vi "test_read-nmea-data2.vi"() -> ()   [LabVIEW 2019] (continued)
,E,2.703,238.94,250720,,,A,V*0C\n\t\n15:14:55.25\tF9P\t$GNVTG,238.94,T,,M,2.703,N,5.005,K,A*21\n\t\n15:14:55.27\tF9P\t$GNGGA,061457.00,3723.60262,N,12656.95923,E,1,12,0.72,45.1,M,18.5,M,,*7E\n\t\n15:14:55.29\tF9P\t$GNGSA,A,3,12,06,19,05,17,09,04,02,,,,,1.24,0.72,1.01,1*02\n\t\n15:14:55.31\tF9P\t$GNGSA,A,3,85,70,71,84,,,,,,,,,1.24,0.72,1.01,2*00\n\t\n15:14:55.33\tF9P\t$GNGSA,A,3,36,19,11,04,09,12,,,,,,,1.24,0.72,1.01,3*02\n\t\n15:14:55.35\tF9P\t$GNGSA,A,3,14,11,33,,,,,,,,,,1.24,0.72,1.01,4*03\n\t\n15:14:55.37\tF9P\t$GPGSV,3,1,09,02,56,320,27,04,17,043,29,05,38,248,35,06,64,051,32,1*63\n\t\n15:14:55.39\tF9P\t$GPGSV,3,2,09,09,44,072,37,12,23,275,25,17,32,154,28,19,51,157,26,1*67\n\t\n15:14:55.41\tF9P\t$GPGSV,3,3,09,25,12,306,15,1*58\n\t\n15:14:55.43\tF9P\t$GPGSV,3,1,09,02,56,320,,04,17,043,19,05,38,248,28,06,64,051,28,6*65\n\t\n15:14:55.45\tF9P\t$GPGSV,3,2,09,09,44,072,29,12,23,275,18,17,32,154,17,19,51,157,,6*69\n\t\n15:14:55.47\tF9P\t$GPGSV,3,3,09,25,12,306,,6*5B\n\t\n15:14:55.49\tF9P\t$GLGSV,2,1,08,69,10,031,30,70,70,037,33,71,54,207,34,72,05,210,,1*7E\n\t\n15:14:55.51\tF9P\t$GLGSV,2,2,08,77,01,324,,84,19,123,18,85,69,072,42,86,38,331,,1*7C\n\t\n15:14:55.53\tF9P\t$GLGSV,2,1,08,69,10,031,19,70,70,037,,71,54,207,30,72,05,210,,3*73\n\t\n15:14:55.55\tF9P\t$GLGSV,2,2,08,77,01,324,,84,19,123,21,85,69,072,24,86,38,331,,3*74\n\t\n15:14:55.57\tF9P\t$GAGSV,2,1,08,02,08,296,09,04,67,115,32,09,33,193,26,11,72,001,25,7*72\n\t\n15:14:55.59\tF9P\t$GAGSV,2,2,08,12,39,103,32,19,25,045,34,25,08,248,14,36,27,309,19,7*7E\n\t\n15:14:55.61\tF9P\t$GAGSV,2,1,08,02,08,296,,04,67,115,,09,33,193,,11,72,001,,2*7C\n\t\n15:14:55.63\tF9P\t$GAGSV,2,2,08,12,39,103,,19,25,045,,25,08,248,,36,27,309,,2*70\n\t\n15:14:55.65\tF9P\t$GBGSV,2,1,06,07,,,26,11,48,133,26,14,87,101,30,28,,,23,1*7B\n\t\n15:14:55.67\tF9P\t$GBGSV,2,2,06,33,62,220,33,34,,,25,1*44\n\t\n15:14:55.69\tF9P\t$GBGSV,1,1,03,11,48,133,,14,87,101,30,33,62,220,,3*47\n\t\n15:14:55.71\tF9P\t$GNGLL,3723.60262,N,12656.95923,E,061457.00,A,A*71\n\t\n15:14:55.73\tF9P\t\t\n15:14:55.75\tF9P\t\t\n15:14:55.77\tF9P\t\t\n15:14:55.79\tF9P\t\t\n15:14:55.81\tF9P\t\t\n15:14:55.83\tF9P\t\t\n15:14:55.85\tF9P\t\t\n15:14:55.87\tF9P\t\t\n15:14:55.89\tF9P\t\t\n15:14:55.91\tF9P\t\t\n15:14:55.93\tF9P\t\t\n15:14:55.95\tF9P\t\t\n15:14:55.97\tF9P\t\t\n15:14:55.99\tF9P\t\t\n15:14:56.01\tF9P\t\t\n15:14:56.03\tF9P\t\t\n15:14:56.05\tF9P\t\t\n15:14:56.07\tF9P\t\t\n15:14:56.09\tF9P\t\t\n15:14:56.11\tF9P\t\t\n15:14:56.13\tF9P\t\t\n15:14:56.15\tF9P\t\t\n15:14:56.17\tF9P\t\t\n15:14:56.19\tF9P\t\t\n15:14:56.21\tF9P\t\t\n15:14:56.23\tF9P\t$GNRMC,061458.00,A,3723.60230,N,12656.95830,E,2.766,236.10,250720,,,A,V*06\n\t\n15:14:56.25\tF9P\t$GNVTG,236.10,T,,M,2.766,N,5.123,K,A*25\n\t\n15:14:56.27\tF9P\t$GNGGA,061458.00,3723.60230,N,12656.95830,E,1,12,0.72,45.0,M,18.5,M,,*74\n\t\n15:14:56.29\tF9P\t$GNGSA,A,3,12,06,19,05,17,09,04,02,,,,,1.24,0.72,1.01,1*02\n\t\n15:14:56.31\tF9P\t$GNGSA,A,3,85,70,71,84,,,,,,,,,1.24,0.72,1.01,2*00\n\t\n15:14:56.33\tF9P\t$GNGSA,A,3,36,19,11,04,09,12,,,,,,,1.24,0.72,1.01,3*02\n\t\n15:14:56.35\tF9P\t$GNGSA,A,3,14,11,33,,,,,,,,,,1.24,0.72,1.01,4*03\n\t\n15:14:56.37\tF9P\t$GPGSV,3,1,09,02,56,320,25,04,17,043,28,05,38,248,36,06,64,051,28,1*68\n\t\n15:14:56.39\tF9P\t$GPGSV,3,2,09,09,44,072,38,12,23,275,24,17,32,154,27,19,51,157,26,1*66\n\t\n15:14:56.41\tF9P\t$GPGSV,3,3,09,25,12,306,14,1*59\n\t\n15:14:56.43\tF9P\t$GPGSV,3,1,09,02,56,320,,04,17,043,19,05,38,248,32,06,64,051,33,6*64\n\t\n15:14:56.45\tF9P\t$GPGSV,3,2,09,09,44,072,29,12,23,275,17,17,32,154,16,19,51,157,,6*67\n\t\n15:14:56.47\tF9P\t$GPGSV,3,3,09,25,12,306,,6*5B\n\t\n15:14:56.49\tF9P\t$GLGSV,2,1,08,69,10,031,23,70,70,037,31,71,54,207,32,72,05,210,,1*78\n\t\n15:14:56.51\tF9P\t$GLGSV,2,2,08,77,01,324,,84,19,123,16,85,69,072,43,86,38,331,,1*73\n\t\n15:14:56.53\tF9P\t$GLGSV,2,1,08,69,10,031,18,70,70,037,,71,54,207,28,72,05,210,,3*7B\n\t\n15:14:56.55\tF9P\t$GLGSV,2,2,08,77,01,324,,84,19,123,19,85,69,072,24,86,38,331,,3*7F\n\t\n15:14:56.57\tF9P\t$GAGSV,2,1,08,02,08,296,09,04,67,115,34,09,33,193,25,11,72,001,25,7*77\n\t\n15:14:56.59\tF9P\t$GAGSV,2,2,08,12,39,103,33,19,25,045,37,25,08,248,15,36,27,309,21,7*76\n\t\n15:14:56.61\tF9P\t$GAGSV,2,1,08,02,08,296,,04,67,115,,09,33,193,,11,72,001,,2*7C\n\t\n15:14:56.63\tF9P\t$GAGSV,2,2,08,12,39,103,,19,25,045,,25,08,248,,36,27,309,,2*70\n\t\n15:14:56.65\tF9P\t$GBGSV,2,1,06,07,,,25,11,48,133,26,14,87,101,29,28,,,22,1*71\n\t\n15:14:56.67\tF9P\t$GBGSV,2,2,06,33,62,220,30,34,,,24,1*46\n\t\n15:14:56.69\tF9P\t$GBGSV,1,1,03,11,48,133,,14,87,101,31,33,62,220,,3*46\n\t\n15:14:56.71\tF9P\t$GNGLL,3723.60230,N,12656.95830,E,061458.00,A,A*7A\n\t\n15:14:56.73\tF9P\t\t\n15:14:56.75\tF9P\t\t\n15:14:56.77\tF9P\t\t\n15:14:56.79\tF9P\t\t\n15:14:56.81\tF9P\t\t\n15:14:56.83\tF9P\t\t\n15:14:56.85\tF9P\t\t\n15:14:56.87\tF9P\t\t\n15:14:56.89\tF9P\t\t\n15:14:56.91\tF9P\t\t\n15:14:56.93\tF9P\t\t\n15:14:56.95\tF9P\t\t\n15:14:56.97\tF9P\t\t\n15:14:56.99\tF9P\t\t\n15:14:57.01\tF9P\t\t\n15:14:57.03\tF9P\t\t\n15:14:57.05\tF9P\t\t\n15:14:57.07\tF9P\t\t\n15:14:57.09\tF9P\t\t\n15:14:57.11\tF9P\t\t\n15:14:57.13\tF9P\t\t\n15:14:57.15\tF9P\t\t\n15:14:57.17\tF9P\t\t\n15:14:57.19\tF9P\t\t\n15:14:57.21\tF9P\t\t\n15:14:57.23\tF9P\t$GNRMC,061459.00,A,3723.60204,N,12656.95730,E,2.820,238.64,250720,,,A,V*0F\n\t\n15:14:57.25\tF9P\t$GNVTG,238.64,T,,M,2.820,N,5.223,K,A*26\n\t\n15:14:57.27\tF9P\t$GNGGA,061459.00,3723.60204,N,12656.95730,E,1,12,0.69,44.9,M,18.5,M,,*7F\n\t\n15:14:57.29\tF9P\t$GNGSA,A,3,12,06,19,05,17,09,04,02,,,,,1.20,0.69,0.98,1*0D\n\t\n15:14:57.31\tF9P\t$GNGSA,A,3,85,70,71,84,,,,,,,,,1.20,0.69,0.98,2*0F\n\t\n15:14:57.33\tF9P\t$GNGSA,A,3,36,19,11,04,09,12,,,,,,,1.20,0.69,0.98,3*0D\n\t\n15:14:57.35\tF9P\t$GNGSA,A,3,14,11,33,,,,,,,,,,1.20,0.69,0.98,4*0C\n\t\n15:14:57.37\tF9P\t$GPGSV,3,1,09,02,56,320,23,04,17,043,26,05,38,248,36,06,64,051,38,1*61\n\t\n15:14:57.39\tF9P\t$GPGSV,3,2,09,09,44,072,38,12,23,275,25,17,32,154,32,19,51,157,26,1*63\n\t\n15:14:57.41\tF9P\t$GPGSV,3,3,09,25,12,306,14,1*59\n\t\n15:14:57.43\tF9P\t$GPGSV,3,1,09,02,56,320,,04,17,043,19,05,38,248,27,06,64,051,28,6*6A\n\t\n15:14:57.45\tF9P\t$GPGSV,3,2,09,09,44,072,30,12,23,275,16,17,32,154,15,19,51,157,,6*6D\n\t\n15:14:57.47\tF9P\t$GPGSV,3,3,09,25,12,306,,6*5B\n\t\n15:14:57.49\tF9P\t$GLGSV,2,1,08,69,10,031,25,70,70,037,25,71,54,207,30,72,05,210,,1*79\n\t\n15:14:57.51\tF9P\t$GLGSV,2,2,08,77,01,324,,84,19,123,16,85,69,072,39,86,38,331,,1*7E\n\t\n15:14:57.53\tF9P\t$GLGSV,2,1,08,69,10,031,18,70,70,037,,71,54,207,25,72,05,210,,3*76\n\t\n15:14:57.55\tF9P\t$GLGSV,2,2,08,77,01,324,,84,19,123,19,85,69,072,25,86,38,331,,3*7E\n\t\n15:14:57.57\tF9P\t$GAGSV,2,1,08,02,08,296,08,04,67,115,26,09,33,193,26,11,72,001,25,7*76\n\t\n15:14:57.59\tF9P\t$GAGSV,2,2,08,12,39,103,33,19,25,045,32,25,08,248,15,36,27,309,22,7*70\n\t\n15:14:57.61\tF9P\t$GAGSV,2,1,08,02,08,296,,04,67,115,,09,33,193,,11,72,001,,2*7C\n\t\n15:14:57.63\tF9P\t$GAGSV,2,2,08,12,39,103,,19,25,045,27,25,08,248,,36,27,309,,2*75\n\t\n15:14:57.65\tF9P\t$GBGSV,2,1,06,07,,,25,11,48,133,26,14,87,101,29,28,,,22,1*71\n\t\n15:14:57.67\tF9P\t$GBGSV,2,2,06,33,62,220,29,34,,,31,1*4A\n\t\n15:14:57.69\tF9P\t$GBGSV,1,1,03,11,48,133,,14,87,101,26,33,62,220,,3*40\n\t\n15:14:57.71\tF9P\t$GNGLL,3723.60204,N,12656.95730,E,061459.00,A,A*73\n\t\n15:14:57.73\tF9P\t\t\n15:14:57.75\tF9P\t\t\n15:14:57.77\tF9P\t\t\n15:14:57.79\tF9P\t\t\n15:14:57.81\tF9P\t\t\n15:14:57.83\tF9P\t\t\n15:14:57.85\tF9P\t\t\n15:14:57.87\tF9P\t\t\n15:14:57.89\tF9P\t\t\n15:14:57.91\tF9P\t\t\n15:14:57.93\tF9P\t\t\n15:14:57.95\tF9P\t\t\n15:14:57.97\tF9P\t\t\n15:14:57.99\tF9P\t\t\n15:14:58.01\tF9P\t\t\n15:14:58.03\tF9P\t\t\n15:14:58.05\tF9P\t\t\n15:14:58.07\tF9P\t\t\n15:14:58.09\tF9P\t\t\n15:14:58.11\tF9P\t\t\n15:14:58.13\tF9P\t\t\n15:14:58.15\tF9P\t\t\n15:14:58.17\tF9P\t\t\n15:14:58.19\tF9P\t\t\n15:14:58.21\tF9P\t\t\n15:14:58.23\tF9P\t$GNRMC,061500.00,A,3723.60170,N,12656.95647,E,2.802,239.48,250720,,,A,V*0C\n\t\n15:14:58.25\tF9P\t$GNVTG,239.48,T,,M,2.802,N,5.190,K,A*22\n\t\n15:14:58.27\tF9P\t$GNGGA,061500.00,3723.60170,N,12656.95647,E,1,12,0.74,45.2,M,18.5,M,,*75\n\t\n15:14:58.29\tF9P\t$GNGSA,A,3,12,06,19,05,17,09,04,02,,,,,1.25,0.74,1.01,1*05\n\t\n15:14:58.31\tF9P\t$GNGSA,A,3,85,70,71,84,,,,,,,,,1.25,0.74,1.01,2*07\n\t\n15:14:58.33\tF9P\t$GNGSA,A,3,36,19,11,04,09,12,,,,,,,1.25,0.74,1.01,3*05\n\t\n15:14:58.35\tF9P\t$GNGSA,A,3,14,11,33,,,,,,,,,,1.25,0.74,1.01,4*04\n\t\n15:14:58.37\tF9P\t$GPGSV,3,1,09,02,56,320,22,04,17,043,27,05,38,248,36,06,64,051,32,1*6B\n\t\n15:14:58.39\tF9P\t$GPGSV,3,2,09,09,44,072,41,12,23,275,26,17,31,154,28,19,51,157,27,1*67\n\t\n15:14:58.41\tF9P\t$GPGSV,3,3,09,25,12,306,14,1*59\n\t\n15:14:58.43\tF9P\t$GPGSV,3,1,09,02,56,320,,04,17,043,19,05,38,248,29,06,64,051,26,6*6A\n\t\n15:14:58.45\tF9P\t$GPGSV,3,2,09,09,44,072,31,12,23,275,15,17,31,154,16,19,51,157,,6*6F\n\t\n15:14:58.47\tF9P\t$GPGSV,3,3,09,25,12,306,,6*5B\n\t\n15:14:58.49\tF9P\t$GLGSV,2,1,08,69,10,031,26,70,70,037,26,71,54,207,31,72,05,210,,1*78\n\t\n15:14:58.51\tF9P\t$GLGSV,2,2,08,77,01,324,,84,19,123,17,85,69,072,36,86,38,331,,1*70\n\t\n15:14:58.53\tF9P\t$GLGSV,2,1,08,69,10,031,17,70,70,037,,71,54,207,26,72,05,210,,3*7A\n\t\n15:14:58.55\tF9P\t$GLGSV,2,2,08,77,01,324,,84,19,123,18,85,69,072,25,86,38,331,,3*7F\n\t\n15:14:58.57\tF9P\t$GAGSV,2,1,08,02,08,296,06,04,67,115,36,09,33,193,26,11,72,001,23,7*7F\n\t\n15:14:58.59\tF9P\t$GAGSV,2,2,08,12,39,103,36,19,25,045,31,25,08,248,14,36,27,309,23,7*76\n\t\n15:14:58.61\tF9P\t$GAGSV,2,1,08,02,08,296,,04,67,115,,09,33,193,,11,72,001,,2*7C\n\t\n15:14:58.63\tF9P\t$GAGSV,2,2,08,12,39,103,,19,25,045,26,25,08,248,,36,27,309,,2*74\n\t\n15:14:58.65\tF9P\t$GBGSV,2,1,06,07,,,27,11,48,133,25,14,87,101,28,28,,,22,1*71\n\t\n15:14:58.67\tF9P\t$GBGSV,2,2,06,33,62,220,29,34,,,25,1*4F\n\t\n15:14:58.69\tF9P\t$GBGSV,1,1,03,11,48,133,,14,87,101,,33,62,220,,3*44\n\t\n15:14:58.71\tF9P\t$GNGLL,3723.60170,N,12656.95647,E,061500.00,A,A*7F\n\t\n15:14:58.73\tF9P\t\t\n15:14:58.75\tF9P\t\t\n15:14:58.77\tF9P\t\t\n15:14:58.79\tF9P\t\t\n15:14:58.81\tF9P\t\t\n15:14:58.83\tF9P\t\t\n15:14:58.85\tF9P\t\t\n15:14:58.87\tF9P\t\t\n15:14:58.89\tF9P\t\t\n15:14:58.91\tF9P\t\t\n15:14:58.93\tF9P\t\t\n15:14:58.95\tF9P\t\t\n15:14:58.97\tF9P\t\t\n15:14:58.99\tF9P\t\t\n15:14:59.01\tF9P\t\t\n15:14:59.03\tF9P\t\t\n15:14:59.05\tF9P\t\t\n15:14:59.07\tF9P\t\t\n15:14:59.09\tF9P\t\t\n15:14:59.11\tF9P\t\t\n15:14:59.13\tF9P\t\t\n15:14:59.15\tF9P\t\t\n15:14:59.17\tF9P\t\t\n15:14:59.19\tF9P\t\t\n15:14:59.21\tF9P\t\t\n15:14:59.23\tF9P\t$GNRMC,061501.00,A,3723.60149,N,12656.95569,E,2.509,241.32,250720,,,A,V*0C\n\t\n15:14:59.25\tF9P\t$GNVTG,241.32,T,,M,2.509,N,4.647,K,A*2A\n\t\n15:14:59.27\tF9P\t$GNGGA,061501.00,3723.60149,N,12656.95569,E,1,12,0.71,45.5,M,18.5,M,,*73\n\t\n15:14:59.29\tF9P\t$GNGSA,A,3,12,06,19,05,17,09,04,02,,,,,1.21,0.71,0.98,1*05\n\t\n15:14:59.31\tF9P\t$GNGSA,A,3,85,70,71,84,,,,,,,,,1.21,0.71,0.98,2*07\n\t\n15:14:59.33\tF9P\t$GNGSA,A,3,36,19,11,04,09,12,,,,,,,1.21,0.71,0.98,3*05\n\t\n15:14:59.35\tF9P\t$GNGSA,A,3,14,11,33,,,,,,,,,,1.21,0.71,0.98,4*04\n\t\n15:14:59.37\tF9P\t$GPGSV,3,1,09,02,56,320,23,04,17,043,28,05,38,248,34,06,64,051,35,1*60\n\t\n15:14:59.39\tF9P\t$GPGSV,3,2,09,09,44,072,43,12,23,275,26,17,31,154,28,19,51,157,25,1*67\n\t\n15:14:59.41\tF9P\t$GPGSV,3,3,09,25,12,306,13,1*5E\n\t\n15:14:59.43\tF9P\t$GPGSV,3,1,09,02,56,320,,04,17,043,18,05,38,248,30,06,64,051,26,6*63\n\t\n15:14:59.45\tF9P\t$GPGSV,3,2,09,09,44,072,31,12,23,275,16,17,31,154,17,19,51,157,,6*6D\n\t\n15:14:59.47\tF9P\t$GPGSV,3,3,09,25,12,306,,6*5B\n\t\n15:14:59.49\tF9P\t$GLGSV,2,1,08,69,10,031,31,70,70,037,27,71,54,207,31,72,05,210,,1*7F\n\t\n15:14:59.51\tF9P\t$GLGSV,2,2,08,77,01,324,,84,19,123,16,85,69,072,28,86,38,331,,1*7E\n\t\n15:14:59.53\tF9P\t$GLGSV,2,1,08,69,10,031,17,70,70,037,,71,54,207,25,72,05,210,,3*79\n\t\n15:14:59.55\tF9P\t$GLGSV,2,2,08,77,01,324,,84,19,123,17,85,69,072,25,86,38,331,,3*70\n\t\n15:14:59.57\tF9P\t$GAGSV,2,1,08,02,08,296,10,04,67,115,35,09,33,193,27,11,72,001,23,7*7A\n\t\n15:14:59.59\tF9P\t$GAGSV,2,2,08,12,39,103,32,19,25,045,26,25,08,248,13,36,27,309,23,7*73\n\t\n15:14:59.61\tF9P\t$GAGSV,2,1,08,02,08,296,,04,67,115,,09,33,193,,11,72,001,,2*7C\n\t\n15:14:59.63\tF9P\t$GAGSV,2,2,08,12,39,103,,19,25,045,24,25,08,248,,36,27,309,,2*76\n\t\n15:14:59.65\tF9P\t$GBGSV,2,1,06,07,,,28,11,48,133,26,14,87,101,28,28,,,23,1*7C\n\t\n15:14:59.67\tF9P\t$GBGSV,2,2,06,33,62,220,31,34,,,25,1*46\n\t\n15:14:59.69\tF9P\t$GBGSV,1,1,03,11,48,133,,14,87,101,,33,62,220,,3*44\n\t\n15:14:59.71\tF9P\t$GNGLL,3723.60149,N,12656.95569,E,061501.00,A,A*7B\n\t\n15:14:59.73\tF9P\t\t\n15:14:59.75\tF9P\t\t\n15:14:59.77\tF9P\t\t\n15:14:59.79\tF9P\t\t\n15:14:59.81\tF9P\t\t\n15:14:59.83\tF9P\t\t\n15:14:59.85\tF9P\t\t\n15:14:59.87\tF9P\t\t\n15:14:59.89\tF9P\t\t\n15:14:59.91\tF9P\t\t\n15:14:59.93\tF9P\t\t\n15:14:59.95\tF9P\t\t\n15:14:59.97\tF9P\t\t\n15:14:59.99\tF9P\t\t\n15:15:00.01\tF9P\t\t\n15:15:00.03\tF9P\t\t\n15:15:00.05\tF9P\t\t\n15:15:00.07\tF9P\t\t\n15:15:00.09\tF9P\t\t\n15:15:00.11\tF9P\t\t\n15:15:00.13\tF9P\t\t\n15:15:00.15\tF9P\t\t\n15:15:00.17\tF9P\t\t\n15:15:00.19\tF9P\t\t\n15:15:00.21\tF9P\t\t\n15:15:00.23\tF9P\t$GNRMC,061502.00,A,3723.60133,N,12656.95493,E,2.633,248.19,250720,,,A,V*0C\n\t\n15:15:00.25\tF9P\t$GNVTG,248.19,T,,M,2.633,N,4.877,K,A*2D\n\t\n15:15:00.27\tF9P\t$GNGGA,061502.00,3723.60133,N,12656.95493,E,1,12,0.67,45.6,M,18.5,M,,*7D\n\t\n15:15:00.29\tF9P\t$GNGSA,A,3,12,06,19,05,17,09,04,02,,,,,1.18,0.67,0.97,1*07\n\t\n15:15:00.31\tF9P\t$GNGSA,A,3,85,70,71,84,,,,,,,,,1.18,0.67,0.97,2*05\n\t\n15:15:00.33\tF9P\t$GNGSA,A,3,36,19,11,04,09,12,,,,,,,1.18,0.67,0.97,3*07\n\t\n15:15:00.35\tF9P\t$GNGSA,A,3,14,11,33,,,,,,,,,,1.18,0.67,0.97,4*06\n\t\n15:15:00.37\tF9P\t$GPGSV,3,1,09,02,56,320,29,04,17,043,33,05,38,248,35,06,64,051,31,1*65\n\t\n15:15:00.39\tF9P\t$GPGSV,3,2,09,09,44,072,41,12,23,275,32,17,31,154,29,19,51,157,26,1*62\n\t\n15:15:00.41\tF9P\t$GPGSV,3,3,09,25,12,306,13,1*5E\n\t\n15:15:00.43\tF9P\t$GPGSV,3,1,09,02,56,320,,04,17,043,19,05,38,248,24,06,64,051,26,6*67\n\t\n15:15:00.45\tF9P\t$GPGSV,3,2,09,09,44,072,28,12,23,275,16,17,31,154,17,19,51,157,,6*65\n\t\n15:15:00.47\tF9P\t$GPGSV,3,3,09,25,12,306,,6*5B\n\t\n15:15:00.49\tF9P\t$GLGSV,2,1,08,69,10,031,25,70,70,037,26,71,54,207,26,72,05,210,,1*7D\n\t\n15:15:00.51\tF9P\t$GLGSV,2,2,08,77,01,324,,84,19,123,14,85,69,072,33,86,38,331,,1*76\n\t\n15:15:00.53\tF9P\t$GLGSV,2,1,08,69,10,031,17,70,70,037,,71,54,207,23,72,05,210,,3*7F\n\t\n15:15:00.55\tF9P\t$GLGSV,2,2,08,77,01,324,,84,19,123,16,85,69,072,25,86,38,331,,3*71\n\t\n15:15:00.57\tF9P\t$GAGSV,2,1,08,02,08,296,09,04,67,115,33,09,33,193,27,11,72,001,22,7*75\n\t\n15:15:00.59\tF9P\t$GAGSV,2,2,08,12,39,103,27,19,25,045,28,25,08,248,,36,27,309,25,7*7D\n\t\n15:15:00.61\tF9P\t$GAGSV,2,1,08,02,08,296,,04,67,115,,09,33,193,,11,72,001,,2*7C\n\t\n15:15:00.63\tF9P\t$GAGSV,2,2,08,12,39,103,,19,25,045,22,25,08,248,,36,27,309,,2*70\n\t\n15:15:00.65\tF9P\t$GBGSV,2,1,06,07,,,26,11,48,133,26,14,87,101,28,28,,,23,1*72\n\t\n15:15:00.67\tF9P\t$GBGSV,2,2,06,33,62,220,26,34,,,31,1*45\n\t\n15:15:00.69\tF9P\t$GBGSV,1,1,03,11,48,133,,14,87,101,26,33,62,220,,3*40\n\t\n15:15:00.71\tF9P\t$GNGLL,3723.60133,N,12656.95493,E,061502.00,A,A*71\n\t\n15:15:00.73\tF9P\t\t\n15:15:00.75\tF9P\t\t\n15:15:00.77\tF9P\t\t\n15:15:00.79\tF9P\t\t\n15:15:00.81\tF9P\t\t\n15:15:00.83\tF9P\t\t\n15:15:00.85\tF9P\t\t\n15:15:00.87\tF9P\t\t\n15:15:00.89\tF9P\t\t\n15:15:00.91\tF9P\t\t\n15:15:00.93\tF9P\t\t\n15:15:00.95\tF9P\t\t\n15:15:00.97\tF9P\t\t\n15:15:00.99\tF9P\t\t\n15:15:01.01\tF9P\t\t\n15:15:01.03\tF9P\t\t\n15:15:01.05\tF9P\t\t\n15:15:01.07\tF9P\t\t\n15:15:01.09\tF9P\t\t\n15:15:01.11\tF9P\t\t\n15:15:01.13\tF9P\t\t\n15:15:01.15\tF9P\t\t\n15:15:01.17\tF9P\t\t\n15:15:01.19\tF9P\t\t\n15:15:01.21\tF9P\t\t\n15:15:01.23\tF9P\t$GNRMC,061503.00,A,3723.60156,N,12656.95384,E,2.728,260.12,250720,,,A,V*05\n\t\n15:15:01.25\tF9P\t$GNVTG,260.12,T,,M,2.728,N,5.053,K,A*28\n\t\n15:15:01.27\tF9P\t$GNGGA,061503.00,3723.60156,N,12656.95384,E,1,12,0.71,46.0,M,18.5,M,,*7C\n\t\n15:15:01.29\tF9P\t$GNGSA,A,3,12,06,19,05,17,09,04,02,,,,,1.21,0.71,0.98,1*05\n\t\n15:15:01.31\tF9P\t$GNGSA,A,3,85,70,71,84,,,,,,,,,1.21,0.71,0.98,2*07\n\t\n15:15:01.33\tF9P\t$GNGSA,A,3,36,19,11,04,09,12,,,,,,,1.21,0.71,0.98,3*05\n\t\n15:15:01.35\tF9P\t$GNGSA,A,3,14,11,33,,,,,,,,,,1.21,0.71,0.98,4*04\n\t\n15:15:01.37\tF9P\t$GPGSV,3,1,09,02,56,320,26,04,17,043,39,05,38,248,35,06,64,051,32,1*63\n\t\n15:15:01.39\tF9P\t$GPGSV,3,2,09,09,44,072,36,12,23,275,29,17,31,154,29,19,51,157,27,1*69\n\t\n15:15:01.41\tF9P\t$GPGSV,3,3,09,25,12,306,14,1*59\n\t\n15:15:01.43\tF9P\t$GPGSV,3,1,09,02,56,320,,04,17,043,20,05,38,248,26,06,64,051,28,6*61\n\t\n15:15:01.45\tF9P\t$GPGSV,3,2,09,09,44,072,28,12,23,275,15,17,31,154,18,19,51,157,,6*69\n\t\n15:15:01.47\tF9P\t$GPGSV,3,3,09,25,12,306,,6*5B\n\t\n15:15:01.49\tF9P\t$GLGSV,2,1,08,69,10,031,25,70,70,037,32,71,54,207,37,72,05,210,,1*78\n\t\n15:15:01.51\tF9P\t$GLGSV,2,2,08,77,01,324,,84,19,123,14,85,69,072,39,86,38,331,,1*7C\n\t\n15:15:01.53\tF9P\t$GLGSV,2,1,08,69,10,031,19,70,70,037,,71,54,207,25,72,05,210,,3*77\n\t\n15:15:01.55\tF9P\t$GLGSV,2,2,08,77,01,324,,84,19,123,18,85,69,072,26,86,38,331,,3*7C\n\t\n15:15:01.57\tF9P\t$GAGSV,2,1,08,02,08,296,11,04,67,115,30,09,33,193,31,11,72,001,23,7*79\n\t\n15:15:01.59\tF9P\t$GAGSV,2,2,08,12,39,103,27,19,25,045,29,25,08,248,,36,27,309,25,7*7C\n\t\n15:15:01.61\tF9P\t$GAGSV,2,1,08,02,08,296,,04,67,115,,09,33,193,,11,72,001,,2*7C\n\t\n15:15:01.63\tF9P\t$GAGSV,2,2,08,12,39,103,,19,25,045,21,25,08,248,,36,27,309,,2*73\n\t\n15:15:01.65\tF9P\t$GBGSV,2,1,06,07,,,25,11,48,133,26,14,87,101,33,28,,,24,1*7C\n\t\n15:15:01.67\tF9P\t$GBGSV,2,2,06,33,62,220,32,34,,,25,1*45\n\t\n15:15:01.69\tF9P\t$GBGSV,1,1,03,11,48,133,,14,87,101,,33,62,220,,3*44\n\t\n15:15:01.71\tF9P\t$GNGLL,3723.60156,N,12656.95384,E,061503.00,A,A*72\n\t\n15:15:01.73\tF9P\t\t\n15:15:01.75\tF9P\t\t\n15:15:01.77\tF9P\t\t\n15:15:01.79\tF9P\t\t\n15:15:01.81\tF9P\t\t\n15:15:01.83\tF9P\t\t\n15:15:01.85\tF9P\t\t\n15:15:01.87\tF9P\t\t\n15:15:01.89\tF9P\t\t\n15:15:01.91\tF9P\t\t\n15:15:01.93\tF9P\t\t\n15:15:01.95\tF9P\t\t\n15:15:01.97\tF9P\t\t\n15:15:01.99\tF9P\t\t\n15:15:02.01\tF9P\t\t\n15:15:02.03\tF9P\t\t\n15:15:02.05\tF9P\t\t\n15:15:02.07\tF9P\t\t\n15:15:02.09\tF9P\t\t\n15:15:02.11\tF9P\t\t\n15:15:02.13\tF9P\t\t\n15:15:02.15\tF9P\t\t\n15:15:02.17\tF9P\t\t\n15:15:02.19\tF9P\t\t\n15:15:02.21\tF9P\t\t\n15:15:02.23\tF9P\t$GNRMC,061504.00,A,3723.60146,N,12656.95282,E,2.604,257.00,250720,,,A,V*0C\n\t\n15:15:02.25\tF9P\t$GNVTG,257.00,T,,M,2.604,N,4.823,K,A*2E\n\t\n15:15:02.27\tF9P\t$GNGGA,061504.00,3723.60146,N,12656.95282,E,1,12,0.71,45.9,M,18.5,M,,*77\n\t\n15:15:02.29\tF9P\t$GNGSA,A,3,12,06,19,05,17,09,04,02,,,,,1.21,0.71,0.98,1*05\n\t\n15:15:02.31\tF9P\t$GNGSA,A,3,85,70,71,84,,,,,,,,,1.21,0.71,0.98,2*07\n\t\n15:15:02.33\tF9P\t$GNGSA,A,3,36,19,11,04,09,12,,,,,,,1.21,0.71,0.98,3*05\n\t\n15:15:02.35\tF9P\t$GNGSA,A,3,14,11,33,,,,,,,,,,1.21,0.71,0.98,4*04\n\t\n15:15:02.37\tF9P\t$GPGSV,3,1,09,02,56,320,26,04,17,043,37,05,38,248,39,06,64,051,35,1*66\n\t\n15:15:02.39\tF9P\t$GPGSV,3,2,09,09,44,072,35,12,23,275,28,17,31,154,30,19,51,157,32,1*67\n\t\n15:15:02.41\tF9P\t$GPGSV,3,3,09,25,12,306,13,1*5E\n\t\n15:15:02.43\tF9P\t$GPGSV,3,1,09,02,56,320,,04,17,043,21,05,38,248,26,06,64,051,29,6*61\n\t\n15:15:02.45\tF9P\t$GPGSV,3,2,09,09,44,072,28,12,23,275,16,17,31,154,20,19,51,157,,6*61\n\t\n15:15:02.47\tF9P\t$GPGSV,3,3,09,25,12,306,,6*5B\n\t\n15:15:02.49\tF9P\t$GLGSV,2,1,08,69,10,031,26,70,70,037,28,71,54,207,31,72,05,210,,1*76\n\t\n15:15:02.51\tF9P\t$GLGSV,2,2,08,77,01,324,,84,19,123,16,85,69,072,26,86,38,331,,1*70\n\t\n15:15:02.53\tF9P\t$GLGSV,2,1,08,69,10,031,17,70,70,037,,71,54,207,23,72,05,210,,3*7F\n\t\n15:15:02.55\tF9P\t$GLGSV,2,2,08,77,01,324,,84,19,123,21,85,69,072,25,86,38,331,,3*75\n\t\n15:15:02.57\tF9P\t$GAGSV,2,1,08,02,08,296,09,04,67,115,34,09,33,193,31,11,72,001,24,7*73\n\t\n15:15:02.59\tF9P\t$GAGSV,2,2,08,12,39,103,26,19,25,045,29,25,08,248,,36,27,309,24,7*7C\n\t\n15:15:02.61\tF9P\t$GAGSV,2,1,08,02,08,296,,04,67,115,,09,33,193,,11,72,001,,2*7C\n\t\n15:15:02.63\tF9P\t$GAGSV,2,2,08,12,39,103,,19,25,045,21,25,08,248,,36,27,309,,2*73\n\t\n15:15:02.65\t
